vi "LUCS001RT_GPS_RS232_ReadN_Bytes.vi"(7 "NumberOfBytesToRead":u16=3, 8 "error in":errorcluster, 9 "FPGA VI Reference":refnum<k20>) -> (0 "error out":errorcluster, 1 "FPGA VI Reference Out":refnum<k20>, 3 "N-BytesOut":u8[](array[numeric]))   [LabVIEW 2020]
uses:
  <vilib>/rvi/interface/nirviMethod/nirviMethod.xnode
  sbRIO-9612/SourceCodeFPGA/LUCS002FPGA_Main.vi
  SourceCode_Host/SourceCode_Host/FPGA Bitfiles/LUCS002h.lvproj_FPGA Target_LUCS002FPGA_Main.vi.lvbit
  <vilib>/FPGAPlugInAG/sbRIO-9612/niLvFpga_ReadFifo_sbRIO-9612.vi
  <vilib>/rvi/errors/niLvFpgaMergeErrorWithErrorCode.vi
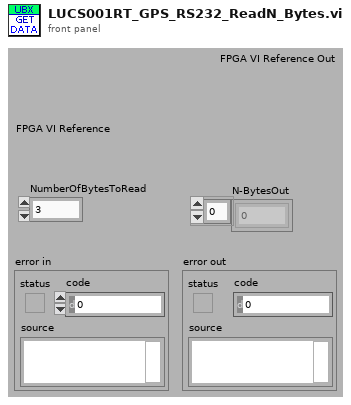
[diagram p1: front panel]
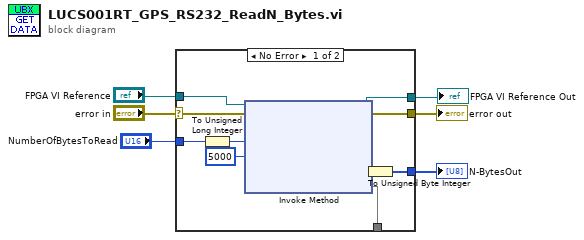
[diagram p0: block diagram]
diagram:
  n1 = case shown="No Error" "error in" {
    selector: "error in" -> [w13 w17]
    tunnel: [w16 _] -> w1
    tunnel: [w15 w17] -> w6
    tunnel: "FPGA VI Reference" -> [w14 _]
    tunnel: [w10 _] -> w4
    tunnel: "NumberOfBytesToRead" -> [w9 _]
    tunnel: [w7 _] -> _
    frame No Error {
      n2 = To Unsigned Long Integer(number=w9) -> (unsigned 32bit integer=w8:u32)
      n3 = xnode "Invoke Method"("FPGA VI Reference In"=w14, "error in"=w13, "Number of Elements"=w8, "Timeout (ms)"=5000) -> ("FPGA VI Reference Out"=w16:refnum<k20>, "error out"=w15:errorcluster, "Data"=w11:void[], "Elements Remaining"=w7)
      n4 = To Unsigned Byte Integer(number=w11) -> (unsigned 8bit integer=w10:u8[])
    }
    frame Error {
    }
  }
  "error out" <- w6
  "N-BytesOut" <- w4
  "FPGA VI Reference Out" <- w1
